vi "BoN_cDAQ Setup_v1.vi"(8 "error in":errorcluster) -> (0 "error out":errorcluster)   [LabVIEW 2022 SP3]
doc: "This VI will perform a self-test of the cDAQ device"
panel:
  in  "stop":bool
  out "Unsuccesful Attempts to connect":i32
  out "Instructional Message":string
  out "Loop Error?":errorcluster
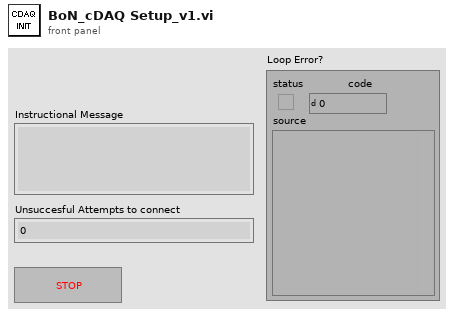
[diagram p1: front panel]
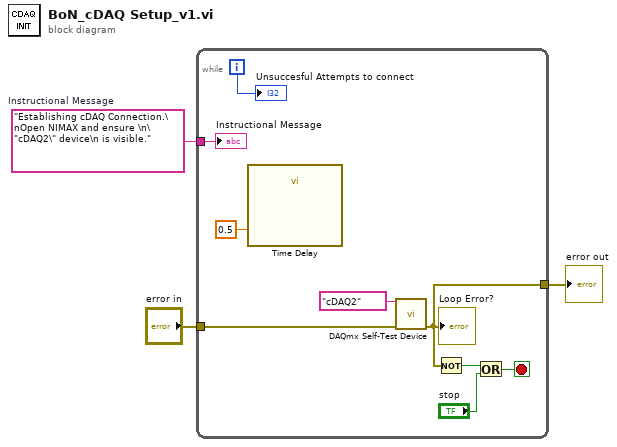
[diagram p0: block diagram]
diagram:
  w1 = "Establishing cDAQ Connection.\nOpen NIMAX and ensure \n\"cDAQ2\" device\n is visible."  # Instructional Message
  n1 = while {
    tunnel: "error in" -> [w12]
    tunnel: [w5] -> w2
    tunnel: w1 -> [w11]
    i -> [w10]
    stop <- w7 stop-if-true
    n2 = call "Time Delay"("Delay Time (s)"=0.5) -> ()  [unwired: 10 in, 1 out]
    n3 = call "DAQmx Self-Test Device.vi"("device in"=tag "cDAQ2", "error in"=w12) -> ("error out"=w5:errorcluster)  [unwired: 13 in]
    "Loop Error?" <- w5
    n4 = Not(x=w5) -> (.not. x?=w9:bool)
    n5 = Or(x=w9, y="stop") -> (x .or. y?=w7:bool)
    "Instructional Message" <- w11
    "Unsuccesful Attempts to connect" <- w10
  }
  "error out" <- w2
